vi "S2C_VLFT10_Proc_SendSwUpdate.vi"(8 "Error In":errorcluster, 11 "Paths":string) -> (0 "Error Out":errorcluster, 3 "Result":string)   [LabVIEW 2015]
uses:
  <vilib>/regexp/Match Regular Expression.xnode
panel:
  in  "PassMatch":string="100\\%[\\s\\S]*?exit"
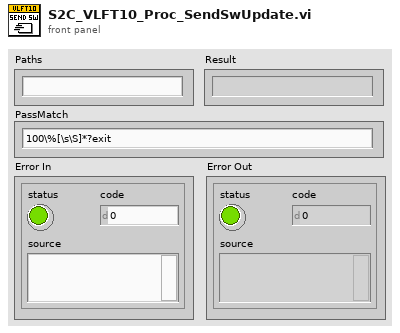
[diagram p1: front panel]
types:
  T1 = cluster{"WinSCP Path":string, "Temp Path":string}
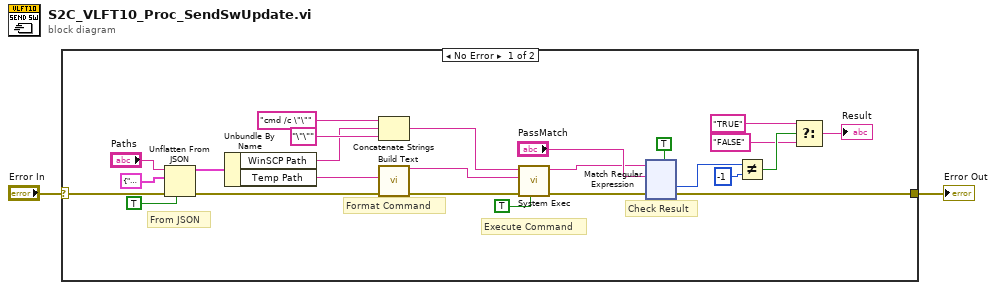
[diagram p0: block diagram]
diagram:
  n1 = case shown="No Error" "Error In" {
    selector: "Error In" -> [w27 w142]
    tunnel: [w22 w142] -> w1
    frame No Error {
      # "Format Command"
      # "From JSON"
      # "Check Result"
      # "Execute Command"
      n2 = Unflatten From JSON(JSON string="Paths", type and defaults=T1 {"WinSCP Path"="", "Temp Path"=""}, default null elements? (F)=TRUE, error in (no error)=w27) -> (value=w6:T1, error out=w12:errorcluster)  [unwired: 3 in]
      n3 = Unbundle By Name(w6) -> ("WinSCP Path"=w5:string, "Temp Path"=w4:string)
      n4 = Concatenate Strings("cmd /c \"\"" ("string"), w5, "\"\"" ("string")) -> (w13:string)
      n5 = call "Build Text"("UploadFilePath"=w4, "error in (no error)"=w12) -> ("Result"=w10:string, "error out"=w11:errorcluster)  [unwired: 12 in]
      n6 = call <vilib>:"System Exec.vi"("run minimized? (F)"=TRUE, "error in (no error)"=w11, "standard input"=w10, "command line"=w13) -> ("error out"=w25:errorcluster, "standard output"=w3:string)  [unwired: 4 in, 2 out]
      n7 = xnode "Match Regular Expression"("input string"=w3, "regular expression"="PassMatch", "error in"=w25, "multiline? (F)"=TRUE) -> ("offset past match"=w21:i32, "error out"=w22:errorcluster)  [unwired: 2 in, 3 out]
      n8 = Not Equal?(x=w21, y=-1) -> (x != y?=w20:bool)
      n9 = Select(t="TRUE", s=w20, f="FALSE") -> (s? t:f=→"Result":string)
    }
    frame Error {
    }
  }
  "Error Out" <- w1
